vi "Reshape_Array_GPS(Subvi).vi"(11 "2차원_GPS_Data":dbl[][](array[numeric])=[[1.0, 2.0, 3.0, 4.0, 5.0], [111.0, 222.0, 333.0, 444.0, 555.0]]) -> (2 "1차원_GPS_Data":dbl[](array[numeric]))   [LabVIEW 2023]
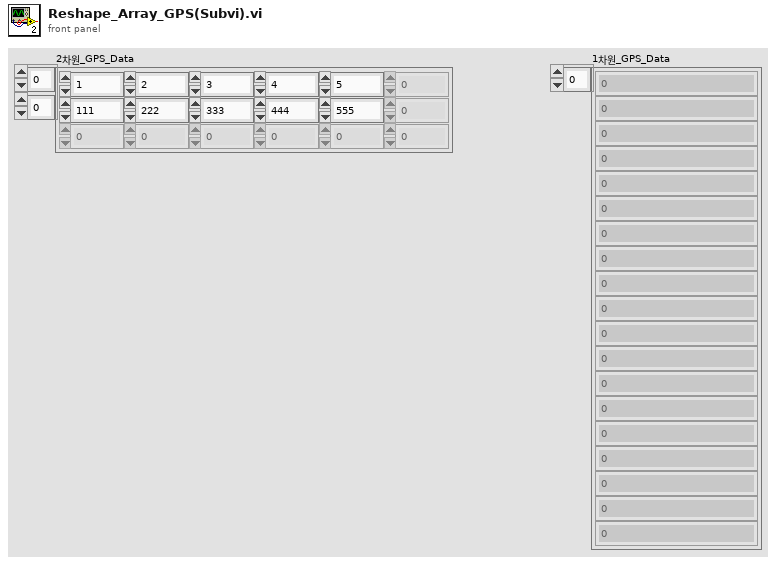
[diagram p1: front panel]
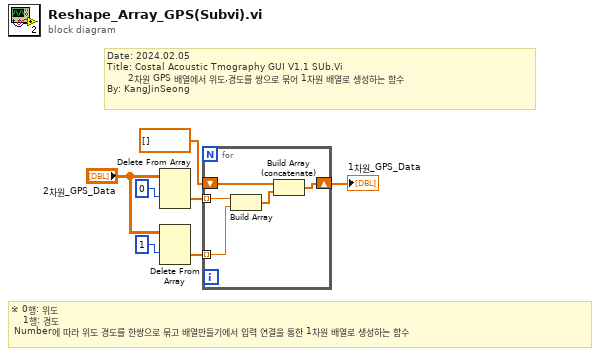
[diagram p0: block diagram]
diagram:
  # "※ 0행: 위도\n    1행: 경도\n Number에 따라 위도 경도를 한쌍으로 묶고 배열만들기에서 입력 연결을 통한 1차원 배열로 생성하는 함수"
  # "Date: 2024.02.05\nTitle: Costal Acoustic Tmography GUI V1.1 SUb.Vi\n       2차원 GPS 배열에서 위도,경도를 쌍으로 묶어 1차원 배열로 생성하는 함수\nBy: KangJinSeong"
  n1 = Delete From Array(array="2차원_GPS_Data", index (row)=0 ("인덱스 (행)")) -> (deleted portion=w3:dbl[])  [unwired: 2 in, 1 out]
  n2 = Delete From Array(array="2차원_GPS_Data", index (row)=1 ("인덱스 (행)")) -> (deleted portion=w6:dbl[])  [unwired: 2 in, 1 out]
  n3 = for {
    tunnel: w6 -> [w11] mode=indexing
    tunnel: w3 -> [w12] mode=indexing
    shift-right: [w8] -> w1
    shift-left: dbl[] [] -> [w10]
    n4 = Build Array(w12, w11) -> (w9:dbl[])
    n5 = Build Array (concatenate)(w10, w9) -> (w8:dbl[])
  }
  "1차원_GPS_Data" <- w1
